vi "Agilent DMM Read Identification.vi"(8 "error in (no error)":errorcluster, 11 "VISA Resource Name":refnum<visa-resource-name>) -> (0 "error out":errorcluster, 1 "Serial Number":string, 2 "Model":string, 3 "dup VISA Resource Name":refnum<visa-resource-name>, 5 "Firmware":string)   [LabVIEW 2011]
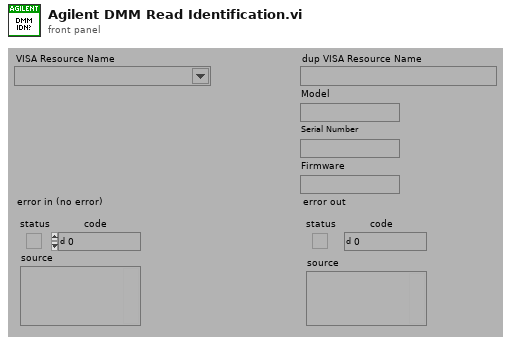
[diagram p1: front panel]
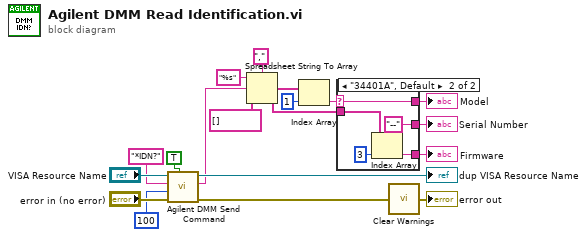
[diagram p0: block diagram]
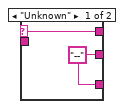
[diagram p2: hidden frame]
diagram:
  n1 = call "Agilent DMM Send Command.vi"("Read? (F)"=TRUE, "error in (no error)"="error in (no error)", "Byte Count"=u32 100 ("byte count"), "Command"="*IDN?", "VISA Resource Name"="VISA Resource Name") -> ("error out"=w5:errorcluster, "Data Read"=w3:string, "dup VISA Resource Name"=→"dup VISA Resource Name":refnum<visa-resource-name>)  [unwired: 4 out]
  n2 = Spreadsheet String To Array(delimiter (Tab)=",", format string="%s", spreadsheet string=w3, array type (2D Dbl)=string[] []) -> (array=w14:string[])
  n3 = Index Array(array=w14, index=1) -> (element=w12:string)
  n4 = case shown="\"34401A\", Default" w12 {
    selector: w12 -> [w20 w25]
    tunnel: [w20 w25] -> w13
    tunnel: w14 -> [_ w23]
    tunnel: [w19 "--"] -> w11
    tunnel: [w19 w22] -> w10
    frame "Unknown" {
      w19 = "--"
    }
    frame "34401A", Default {
      n5 = Index Array(array=w23, index=3) -> (element=w22:string)
    }
  }
  "Model" <- w13
  "Serial Number" <- w11
  "Firmware" <- w10
  n6 = call "Clear Warnings.vi"("error in (no error)"=w5) -> ("error out"=→"error out":errorcluster)
